vi "Move arm.vi"(7 "Description":string, 8 "Command Info In":T2, 10 "Future Positions":T1[](array[typedef]), 11 "Arm Position":T1=enum."Hatch - Ground") -> (0 "Command Info Out":T2)   [LabVIEW 2018]
doc: "This template is useful for immediate subsystem actions that do not need deadband filtering\n\nBe sure to right-click and select New from Template and save with a new command name."
uses:
  <vilib>/Rock Robotics/WPI/Framework/Command Status Info.ctl
  <vilib>/Rock Robotics/WPI/Framework/Completion Status.ctl
  <vilib>/Rock Robotics/WPI/Framework/Completion Notifier.ctl
  Arm Positions.ctl
  Implementation/Arm Setpoints.ctl
  Implementation/Arm Operations.ctl
  Implementation/Arm Published Globals.vi
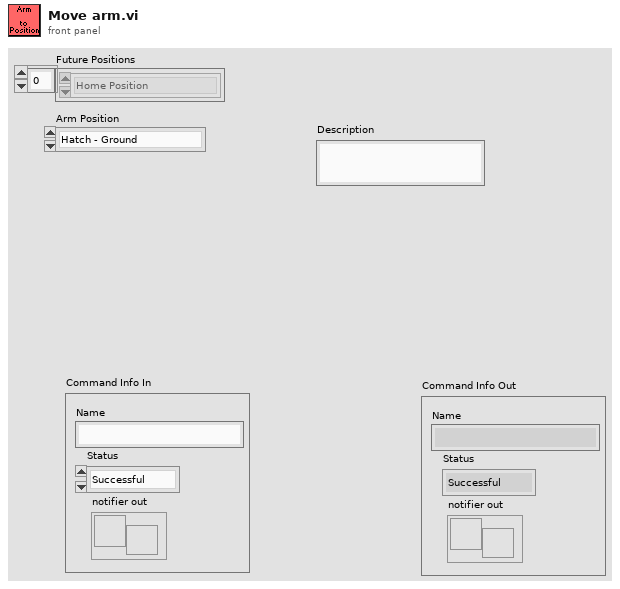
[diagram p1: front panel]
types:
  T1 = typedef "Arm Positions.ctl" = enum16{"Home Position", "Safe Position", "Hatch - Ground", "Hatch - Low", "Hatch - Middle", "High - Safe", "Hatch - High", "Cargo - Low", "Cargo - Middle", "Cargo - High", "Cargo - Loading Station", "Hatch - Loading Station", "Cargo - Ground", "Turret - Left", "Turret - Front", "Turret - Right", "Turret - Back", "Climbing - Forward", "Middle - Safe", "Low - Safe", "Safe Elbow up"}
  T2 = typedef "Command Status Info.ctl" = cluster{"Name":string, "Status":T3, "notifier out":T4}
  T3 = typedef "Completion Status.ctl" = enum16{"Successful", "Aborted", "Incomplete"}
  T4 = typedef "Completion Notifier.ctl" = refnum<notifier>
  T5 = typedef "Arm Setpoints.ctl" = cluster{"Operation":T6, "Turret Setpoint":dbl, "Shoulder Setpoint":dbl, "Elbow Setpoint":dbl, "Wrist Setpoint":dbl, "Axis Enabled":bool[], "Future Positions":T1[]}
  T6 = typedef "Arm Operations.ctl" = enum16{"Reserve", "Read Current", "Immediate", "Immediate Champ", "Move arm to position", "Reset Encoders", "Reset Turret", "Reset Shoulder", "Reset Elbow", "Reset Wrist", "Hold Encoder Counts"}
  T7 = cluster{"Current Command":T5, "Command Timing":cluster{"Start Time (ms)":u32, "Iterations":i32}, "Command Arguments":cluster{"Command Info":T2, "Description":string, "Default Command":T5, "queue out":refnum<queue>, "Subsystem Name":string}}
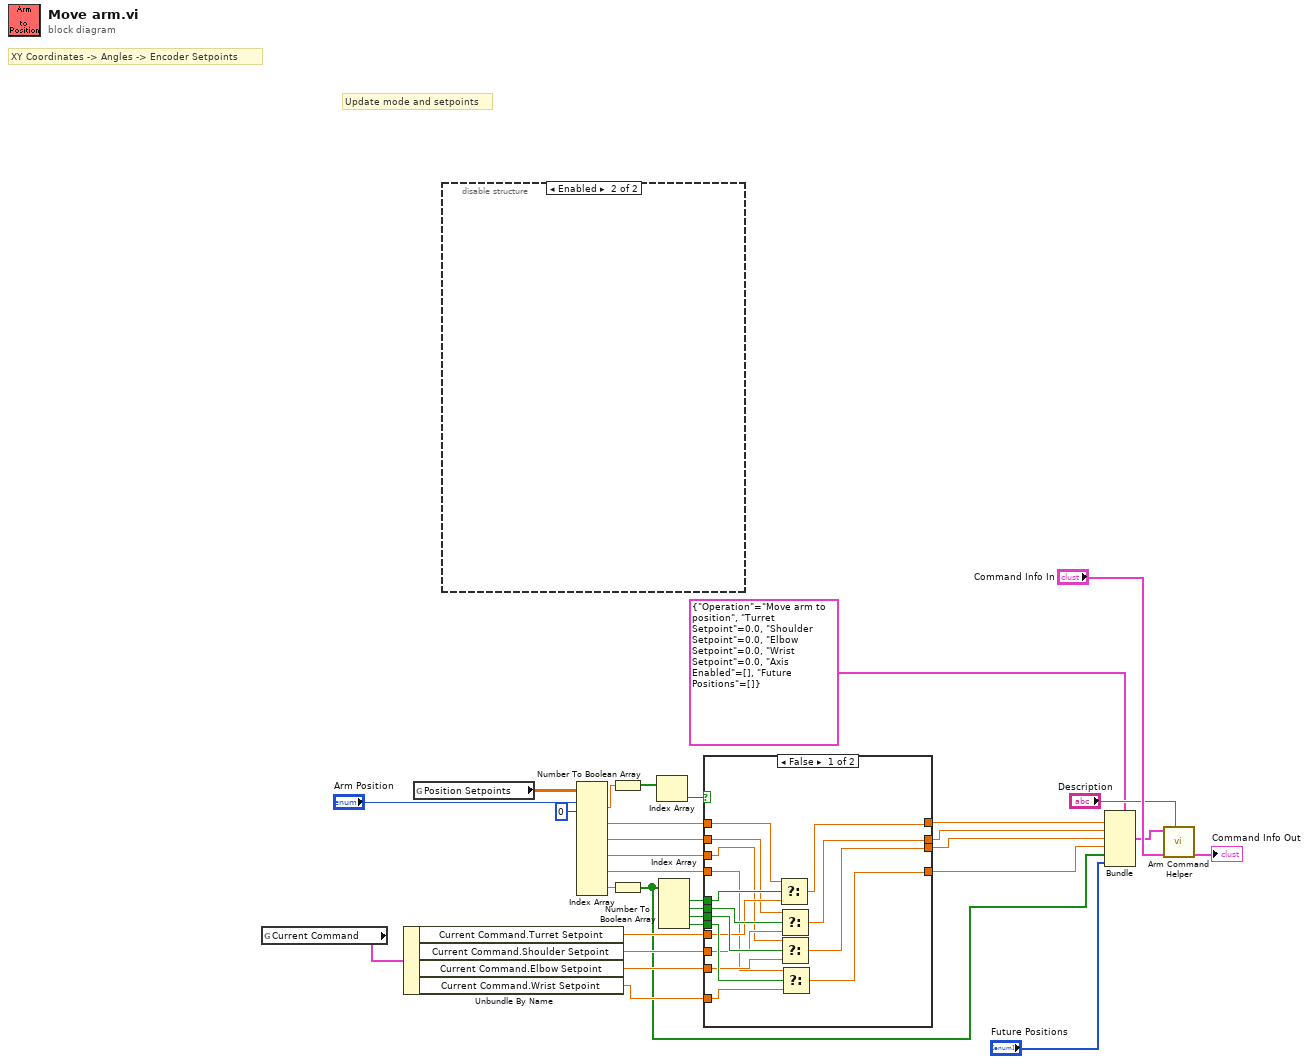
[diagram p0: block diagram]
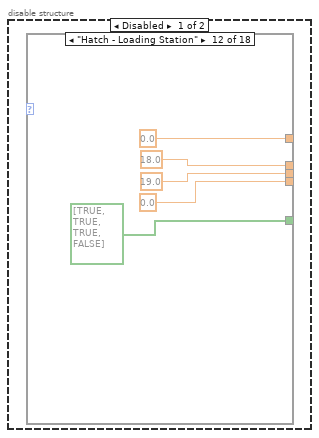
[diagram p2: hidden frame]
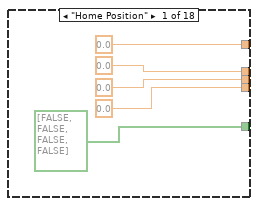
[diagram p3: hidden frame]
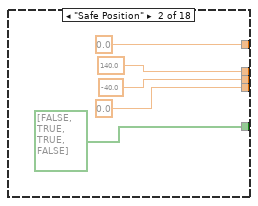
[diagram p4: hidden frame]
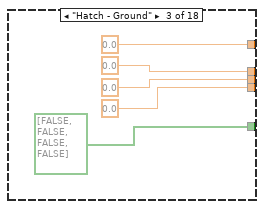
[diagram p5: hidden frame]
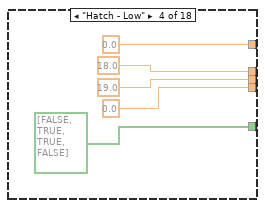
[diagram p6: hidden frame]
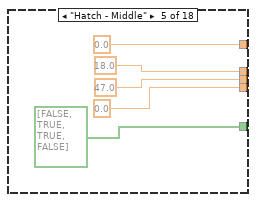
[diagram p7: hidden frame]
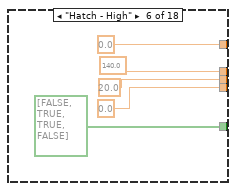
[diagram p8: hidden frame]
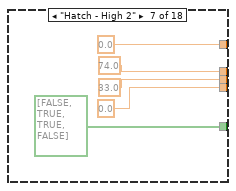
[diagram p9: hidden frame]
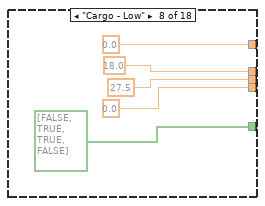
[diagram p10: hidden frame]
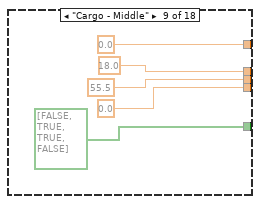
[diagram p11: hidden frame]
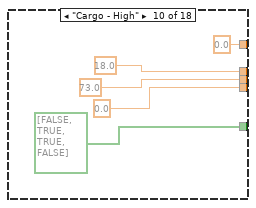
[diagram p12: hidden frame]
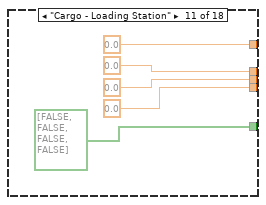
[diagram p13: hidden frame]
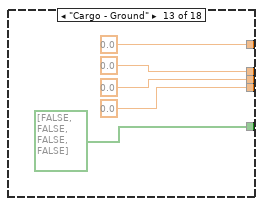
[diagram p14: hidden frame]
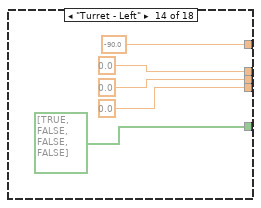
[diagram p15: hidden frame]
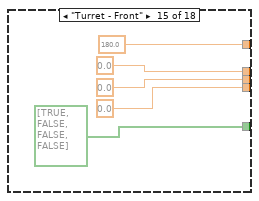
[diagram p16: hidden frame]
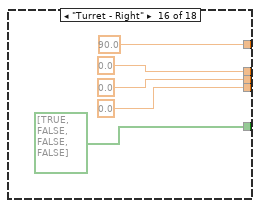
[diagram p17: hidden frame]
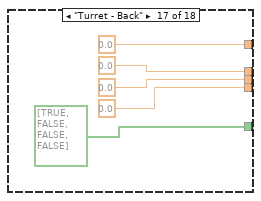
[diagram p18: hidden frame]
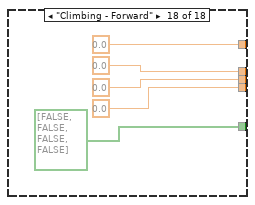
[diagram p19: hidden frame]
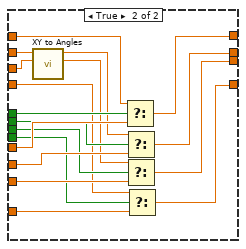
[diagram p20: hidden frame]
diagram:
  # "XY Coordinates -> Angles -> Encoder Setpoints"
  # "Update mode and setpoints"
  n1 = global read "Arm Published Globals.vi" "Current Command"() -> (w10:T7)
  n2 = Unbundle By Name(w10) -> ("Current Command.Turret Setpoint"=w5:dbl, "Current Command.Shoulder Setpoint"=w4:dbl, "Current Command.Elbow Setpoint"=w3:dbl, "Current Command.Wrist Setpoint"=w2:dbl)
  n3 = global read "Arm Published Globals.vi" "Position Setpoints"() -> (w26:dbl[][])
  n4 = disable-structure shown="Enabled" {
    frame Disabled {
      n5 = case shown="\"Hatch - Loading Station\"" {
        selector: _ -> [_ _ _ _ _ _ _ _ _ _ _ _ _ _ _ _ _ _]
        tunnel: [0.0 0.0 0.0 0.0 0.0 0.0 0.0 0.0 0.0 0.0 0.0 0.0 0.0 -90.0 180.0 90.0 0.0 0.0] -> _
        tunnel: [0.0 140.0 0.0 18.0 18.0 140.0 74.0 18.0 18.0 18.0 0.0 18.0 0.0 0.0 0.0 0.0 0.0 0.0] -> _
        tunnel: [0.0 0.0 0.0 0.0 0.0 0.0 0.0 0.0 0.0 0.0 0.0 0.0 0.0 0.0 0.0 0.0 0.0 0.0] -> _
        tunnel: [0.0 -40.0 0.0 19.0 47.0 20.0 33.0 27.5 55.5 73.0 0.0 19.0 0.0 0.0 0.0 0.0 0.0 0.0] -> _
        tunnel: [bool[] [FALSE, FALSE, FALSE, FALSE] ("Axis Enabled") bool[] [FALSE, TRUE, TRUE, FALSE] ("Axis Enabled") bool[] [FALSE, FALSE, FALSE, FALSE] ("Axis Enabled") bool[] [FALSE, TRUE, TRUE, FALSE] ("Axis Enabled") bool[] [FALSE, TRUE, TRUE, FALSE] ("Axis Enabled") bool[] [FALSE, TRUE, TRUE, FALSE] ("Axis Enabled") bool[] [FALSE, TRUE, TRUE, FALSE] ("Axis Enabled") bool[] [FALSE, TRUE, TRUE, FALSE] ("Axis Enabled") bool[] [FALSE, TRUE, TRUE, FALSE] ("Axis Enabled") bool[] [FALSE, TRUE, TRUE, FALSE] ("Axis Enabled") bool[] [FALSE, FALSE, FALSE, FALSE] ("Axis Enabled") bool[] [TRUE, TRUE, TRUE, FALSE] ("Axis Enabled") bool[] [FALSE, FALSE, FALSE, FALSE] ("Axis Enabled") bool[] [TRUE, FALSE, FALSE, FALSE] ("Axis Enabled") bool[] [TRUE, FALSE, FALSE, FALSE] ("Axis Enabled") bool[] [TRUE, FALSE, FALSE, FALSE] ("Axis Enabled") bool[] [TRUE, FALSE, FALSE, FALSE] ("Axis Enabled") bool[] [FALSE, FALSE, FALSE, FALSE] ("Axis Enabled")] -> _
        frame "Home Position" {
        }
        frame "Safe Position" {
        }
        frame "Hatch - Ground" {
        }
        frame "Hatch - Low" {
        }
        frame "Hatch - Middle" {
        }
        frame "Hatch - High" {
        }
        frame "Hatch - High 2" {
        }
        frame "Cargo - Low" {
        }
        frame "Cargo - Middle" {
        }
        frame "Cargo - High" {
        }
        frame "Cargo - Loading Station" {
        }
        frame "Hatch - Loading Station" {
        }
        frame "Cargo - Ground" {
        }
        frame "Turret - Left" {
        }
        frame "Turret - Front" {
        }
        frame "Turret - Right" {
        }
        frame "Turret - Back" {
        }
        frame "Climbing - Forward" {
        }
      }
    }
    frame Enabled {
    }
  }
  n6 = Index Array(array=w26, index (row) #1="Arm Position", index (col) #1=0 ("disabled index (col)")) -> (element #1=w23:dbl, element #2=w19:dbl, element #3=w18:dbl, element #4=w17:dbl, element #5=w16:dbl, element #6=w21:dbl)  [unwired: 10 in]
  n7 = Number To Boolean Array(number=w23) -> (Boolean array=w22:bool[])
  n8 = Number To Boolean Array(number=w21) -> (Boolean array=w1:bool[])
  n9 = Index Array(array=w22) -> (element=w20:bool)  [unwired: 1 in]
  n10 = Index Array(array=w1) -> (element #1=w9:bool, element #2=w8:bool, element #3=w7:bool, element #4=w6:bool)  [unwired: 4 in]
  n11 = case shown="False" w20 {
    tunnel: w19 -> [w128 w140]
    tunnel: w18 -> [w126 w155]
    tunnel: w17 -> [w125 w154]
    tunnel: [w127 w138] -> w13
    tunnel: [w124 w143] -> w12
    tunnel: w16 -> [w122 w144]
    tunnel: [w123 w145] -> w11
    tunnel: [w129 w139] -> w15
    tunnel: w9 -> [w137 w153]
    tunnel: w8 -> [w136 w151]
    tunnel: w7 -> [w135 w147]
    tunnel: w6 -> [w134 w146]
    tunnel: w5 -> [w130 w152]
    tunnel: w4 -> [w131 w150]
    tunnel: w3 -> [w132 w149]
    tunnel: w2 -> [w133 w148]
    frame False {
      n12 = Select(t=w128, s=w137, f=w130) -> (s? t:f=w129:dbl)
      n13 = Select(t=w126, s=w136, f=w131) -> (s? t:f=w127:dbl)
      n14 = Select(t=w125, s=w135, f=w132) -> (s? t:f=w124:dbl)
      n15 = Select(t=w122, s=w134, f=w133) -> (s? t:f=w123:dbl)
    }
    frame True {
      n16 = call "XY to Angles.vi"("Z Target Position"=w154, "X Target Position"=w155) -> ("Elbow Angle"=w142:dbl, "Shoulder Angle"=w141:dbl)  [unwired: 8 in]
      n17 = Select(t=w140, s=w153, f=w152) -> (s? t:f=w139:dbl)
      n18 = Select(t=w141, s=w151, f=w150) -> (s? t:f=w138:dbl)
      n19 = Select(t=w142, s=w147, f=w149) -> (s? t:f=w143:dbl)
      n20 = Select(t=w144, s=w146, f=w148) -> (s? t:f=w145:dbl)
    }
  }
  n21 = Bundle(cluster=T5 {"Operation"=enum."Move arm to position", "Turret Setpoint"=0.0, "Shoulder Setpoint"=0.0, "Elbow Setpoint"=0.0, "Wrist Setpoint"=0.0, "Axis Enabled"=[], "Future Positions"=[]} ("SubSystem Data"), "Turret Setpoint"=w15, "Shoulder Setpoint"=w13, "Elbow Setpoint"=w12, "Wrist Setpoint"=w11, "Axis Enabled"=w1, "Future Positions"="Future Positions") -> (w27:T5)  [unwired: 1 in]
  n22 = call "Arm Command Helper.vi"("Description"="Description", "Command Info In"="Command Info In", "SubSystem Data"=w27) -> ("Command Info Out"=→"Command Info Out":T2)  [unwired: 6 in, 2 out]
